vi "test Parse Boolean.vi"() -> (0 "error out":errorcluster, 2 "pass?":bool)   [LabVIEW 2019, in "RESP3 Tests.lvlib"]
uses:
  RESP3/RESP3 Parser/RESP3 Parser.lvclass
  RESP3/types/RESP3 Type.ctl
  RESP3/types/RESP3 data type attribute.vi
  RESP3 Tests.lvlib
  RESP3/RESP3.lvlib
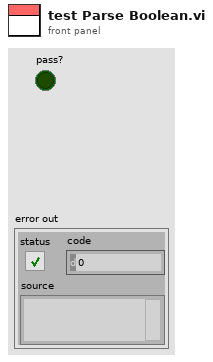
[diagram p1: front panel]
types:
  T1 = typedef "RESP3.lvlib/RESP3 Type.ctl" = enum8{"<0x00>", "<0x01>", "<0x02>", "<0x03>", "<0x04>", "<0x05>", "<0x06>", "<0x07>", "<0x08>", "<0x09>", "<0x0A>", "<0x0B>", "<0x0C>", "<0x0D>", "<0x0E>", "<0x0F>", "<0x10>", "<0x11>", "<0x12>", "<0x13>", "<0x14>", "<0x15>", "<0x16>", "<0x17>", "<0x18>", "<0x19>", "<0x1A>", "<0x1B>", "<0x1C>", "<0x1D>", "<0x1E>", "<0x1F>", "\" \"", "BLOB ERROR", "\"\"\"", "BOOLEAN", "BLOB", "MAP", "\"&\"", "\"'\"", "BIG NUMBER", "\")\"", "ARRAY", "STRING", "DOUBLE", "ERROR", "END", "\"/\"", "\"0\"", "\"1\"", "\"2\"", "\"3\"", "\"4\"", "\"5\"", "\"6\"", "\"7\"", "\"8\"", "\"9\"", "INTEGER", "STREAM", "\"<\"", "VERBATIM STRING", "PUSH", "\"?\"", "\"@\"", "\"A\"", "\"B\"", "\"C\"", "\"D\"", "\"E\"", "\"F\"", "\"G\"", "\"H\"", "\"I\"", "\"J\"", "\"K\"", "\"L\"", "\"M\"", "\"N\"", "\"O\"", "\"P\"", "\"Q\"", "\"R\"", "\"S\"", "\"T\"", "\"U\"", "\"V\"", "\"W\"", "\"X\"", "\"Y\"", "\"Z\"", "\"[\"", "\"\\\"", "\"]\"", "\"^\"", "NULL", "\"`\"", "\"a\"", "\"b\"", "\"c\"", "\"d\"", "\"e\"", "\"f\"", "\"g\"", "\"h\"", "\"i\"", "\"j\"", "\"k\"", "\"l\"", "\"m\"", "\"n\"", "\"o\"", "\"p\"", "\"q\"", "\"r\"", "\"s\"", "\"t\"", "\"u\"", "\"v\"", "\"w\"", "\"x\"", "\"y\"", "\"z\"", "\"{\"", "ATTRIBUTES", "\"}\"", "SET", "<0x7F>", "<0x80>", "<0x81>", "<0x82>", "<0x83>", "<0x84>", "<0x85>", "<0x86>", "<0x87>", "<0x88>", "<0x89>", "<0x8A>", "<0x8B>", "<0x8C>", "<0x8D>", "<0x8E>", "<0x8F>", "<0x90>", "<0x91>", "<0x92>", "<0x93>", "<0x94>", "<0x95>", "<0x96>", "<0x97>", "<0x98>", "<0x99>", "<0x9A>", "<0x9B>", "<0x9C>", "<0x9D>", "<0x9E>", "<0x9F>", "<0xA0>", "<0xA1>", "<0xA2>", "<0xA3>", "<0xA4>", "<0xA5>", "<0xA6>", "<0xA7>", "<0xA8>", "<0xA9>", "<0xAA>", "<0xAB>", "<0xAC>", "<0xAD>", "<0xAE>", "<0xAF>", "<0xB0>", "<0xB1>", "<0xB2>", "<0xB3>", "<0xB4>", "<0xB5>", "<0xB6>", "<0xB7>", "<0xB8>", "<0xB9>", "<0xBA>", "<0xBB>", "<0xBC>", "<0xBD>", "<0xBE>", "<0xBF>", "<0xC0>", "<0xC1>", "<0xC2>", "<0xC3>", "<0xC4>", "<0xC5>", "<0xC6>", "<0xC7>", "<0xC8>", "<0xC9>", "<0xCA>", "<0xCB>", "<0xCC>", "<0xCD>", "<0xCE>", "<0xCF>", "<0xD0>", "<0xD1>", "<0xD2>", "<0xD3>", "<0xD4>", "<0xD5>", "<0xD6>", "<0xD7>", "<0xD8>", "<0xD9>", "<0xDA>", "<0xDB>", "<0xDC>", "<0xDD>", "<0xDE>", "<0xDF>", "<0xE0>", "<0xE1>", "<0xE2>", "<0xE3>", "<0xE4>", "<0xE5>", "<0xE6>", "<0xE7>", "<0xE8>", "<0xE9>", "<0xEA>", "<0xEB>", "<0xEC>", "<0xED>", "<0xEE>", "<0xEF>", "<0xF0>", "<0xF1>", "<0xF2>", "<0xF3>", "<0xF4>", "<0xF5>", "<0xF6>", "<0xF7>", "<0xF8>", "<0xF9>", "<0xFA>", "<0xFB>", "<0xFC>", "<0xFD>", "<0xFE>"}
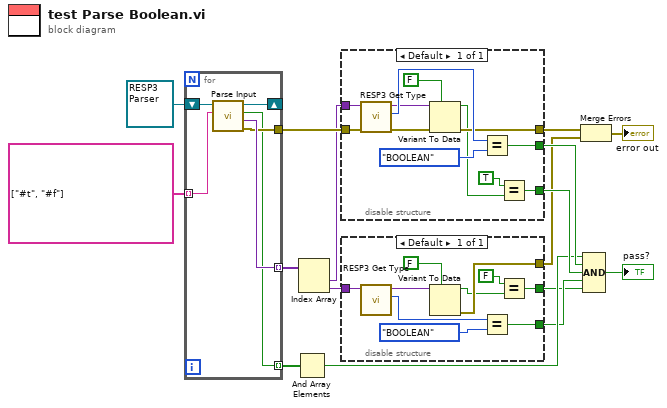
[diagram p0: block diagram]
diagram:
  n1 = for {
    shift-right: [w21] -> _
    shift-left: refnum<class "RESP3 Parser.lvclass"> refnum ("RESP3.lvlib:RESP3 Parser.lvclass") -> [w22]
    tunnel: string[] ["#t", "#f"] -> [w20] mode=indexing
    tunnel: [w19] -> w11 mode=indexing
    tunnel: [w18] -> w10
    tunnel: [w17] -> w8 mode=indexing
    n2 = call-dynamic "Parse Input.vi"("input line"=w20, "RESP3 Parser in"=w22) -> ("error out"=w18:errorcluster, "RESP3 Value"=w19:variant, "finished?"=w17:bool, "RESP3 Parser out"=w21:refnum<class "RESP3 Parser.lvclass">)  [unwired: 6 in]
  }
  n3 = And Array Elements(Boolean array=w8) -> (logical AND=w7:bool)
  n4 = Index Array(array=w11) -> (element #1=w6:variant, element #2=w5:variant)  [unwired: 2 in]
  n5 = disable-structure shown="Default" {
    disable-tunnel: [w31] -> w14
    disable-tunnel: [w24] -> w13
    disable-tunnel: w6 -> [w29]
    disable-tunnel: w10 -> [w28]
    disable-tunnel: [w27] -> w9
    frame Enabled {
      n6 = call "RESP3 Get Type.vi"("RESP3 Value in"=w29) -> ("RESP3 Type"=w32:T1, "RESP3 Value out"=w30:variant)  [unwired: 7 in, 2 out]
      n7 = Variant To Data(error in=w28, type=FALSE, Variant=w30) -> (data=w25:bool, error out=w27:errorcluster)
      n8 = Equal?(x=w32, y=RESP3_Type."BOOLEAN") -> (x = y?=w31:bool)
      n9 = Equal?(x=TRUE, y=w25) -> (x = y?=w24:bool)
    }
  }
  n10 = disable-structure shown="Default" {
    disable-tunnel: [w41] -> w4
    disable-tunnel: [w36] -> w3
    disable-tunnel: [w39] -> w1
    disable-tunnel: w5 -> [w34]
    frame Enabled {
      n11 = call "RESP3 Get Type.vi"("RESP3 Value in"=w34) -> ("RESP3 Type"=w42:T1, "RESP3 Value out"=w40:variant)  [unwired: 7 in, 2 out]
      n12 = Variant To Data(type=FALSE, Variant=w40) -> (data=w37:bool, error out=w39:errorcluster)  [unwired: 1 in]
      n13 = Equal?(x=w42, y=RESP3_Type."BOOLEAN") -> (x = y?=w41:bool)
      n14 = Equal?(x=FALSE, y=w37) -> (x = y?=w36:bool)
    }
  }
  n15 = Merge Errors(w9, w1) -> (→"error out":errorcluster)
  n16 = Compound Arithmetic op=AND(w7, w14, w13, w4, w3) -> (→"pass?":bool)
